vi "InputRegisters.vi"(5 "Input Registers":u16[](array[numeric])) -> (0 "光敏传感器":u16, 1 "内部温度传感器":dbl, 2 "电压(PA5-ADC)":dbl)   [LabVIEW 2013]
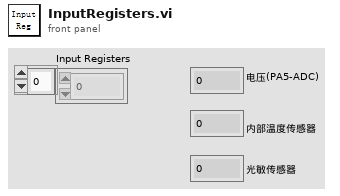
[diagram p1: front panel]
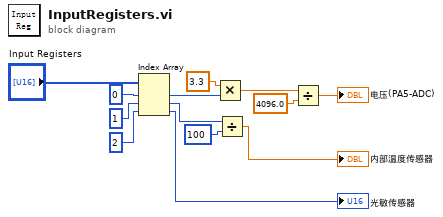
[diagram p0: block diagram]
diagram:
  n1 = Index Array(array="Input Registers", index #1=0 ("索引"), index #2=1 ("索引"), index #3=2 ("索引")) -> (element #1=w7:u16, element #2=w3:u16, element #3=→"光敏传感器":u16)
  n2 = Multiply(x=3.3, y=w7) -> (x*y=w6:dbl)
  n3 = Divide(x=w3, y=u16 100) -> (x/y=→"内部温度传感器":dbl)
  n4 = Divide(x=w6, y=4096.0) -> (x/y=→"电压(PA5-ADC)":dbl)
